vi "Expert_DescriptionError.vi"(4 "Error IN Toolkit":i32, 5 "Error IN LabVIEW":errorcluster) -> (18 "Error_msg":string, 19 "Error OUT LabVIEW":errorcluster)   [LabVIEW 2018]
doc: "Informs in detail about what error in the Toolkit has occurred. It receives the error from a VI that is using the DLL."
panel:
  out "Error OUT Toolkit":i32
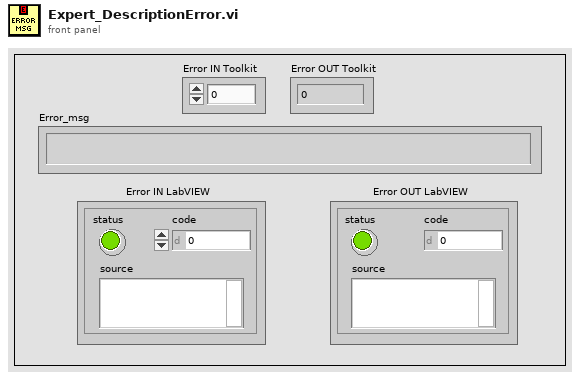
[diagram p1: front panel]
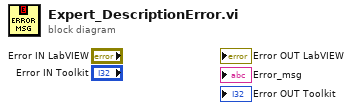
[diagram p0: block diagram]
diagram:
